vi "NAMEdll.vi"(7 "ln3":i32, 8 "error in (no error)":errorcluster, 9 "ln2":i32, 10 "ln1":i32, 11 "Mixure Cluster in":T1={"Mixture Name"="R410A", "Molecular weight (g/mol)"=72.5854142406597, "Critical temperature (K)"=343.606231592265, "Critical Pressure (kPa)"=4813.60652781276, "Critical Density (mol/L)"=0.0, "# Components"=2, "Fluid File Paths"=[path "C:/Program Files (x86)/National Instruments/LabVIEW 2015/user.lib/REFPROP/fluids/R32.FLD", path "C:/Program Files (x86)/National Instruments/LabVIEW 2015/user.lib/REFPROP/fluids/R125.FLD"], "Component molar fractions"=[0.697614699375863, 0.302385300624138], "Refprop Main Directory"=path "C:/Program Files (x86)/National Instruments/LabVIEW 2015/user.lib/REFPROP", "DLL Version Number"=0.0}) -> (0 "error out":errorcluster, 3 "name out":string)   [LabVIEW 2015]
doc: "subroutine NAMEdll(icomp, hnam, hn80, hcasn, hnam_length, hn80_length, hcasn_length)\nProvides name information for the specified component.\n\nINPUTS:\n icomp ::Component number in mixture; 1 for pure fluid\n ln1 :: length of variable hnam (default: 12)\n ln2 :: length of variable hn80 (default: 80)\n ln3 :: length of variable hcasn (default: 12)\n\nOUTPUTS:\nhnam :: Component name (character*12)\nhn80 :: Component name - long form (character*80) To return the file name used when SETUP\n was called (without path), send -icomp. If path is also needed, use PASSCMN.\nhcasn :: ID (Chemical Abstracts Service) number (character*12)"
uses:
  Ctl/Mixture Composition cluster_d.ctl
  REFPROP.dll
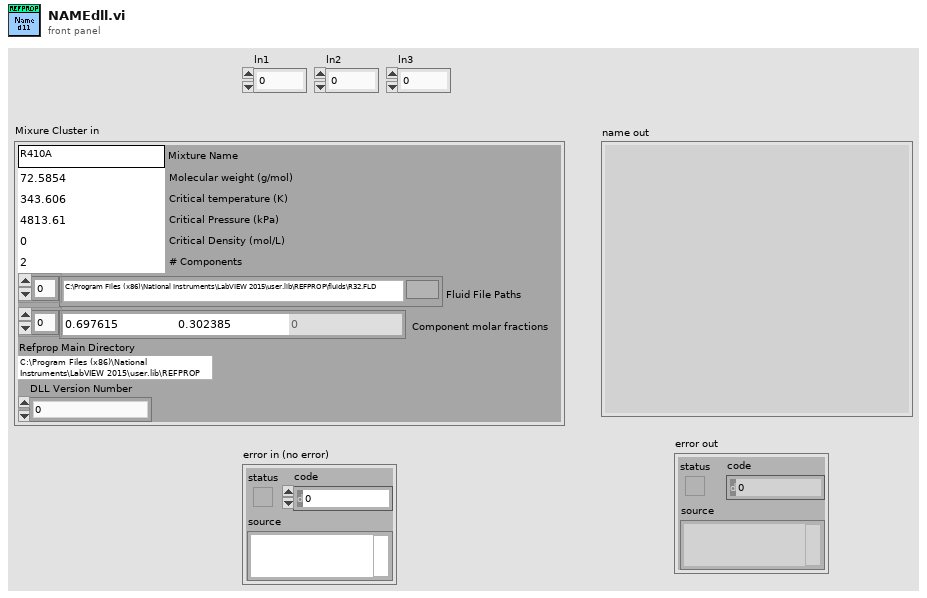
[diagram p1: front panel]
types:
  T1 = typedef "Mixture Composition cluster_d.ctl" = cluster{"Mixture Name":string, "Molecular weight (g/mol)":dbl, "Critical temperature (K)":dbl, "Critical Pressure (kPa)":dbl, "Critical Density (mol/L)":dbl, "# Components":i32, "Fluid File Paths":path[], "Component molar fractions":dbl[], "Refprop Main Directory":path, "DLL Version Number":dbl}
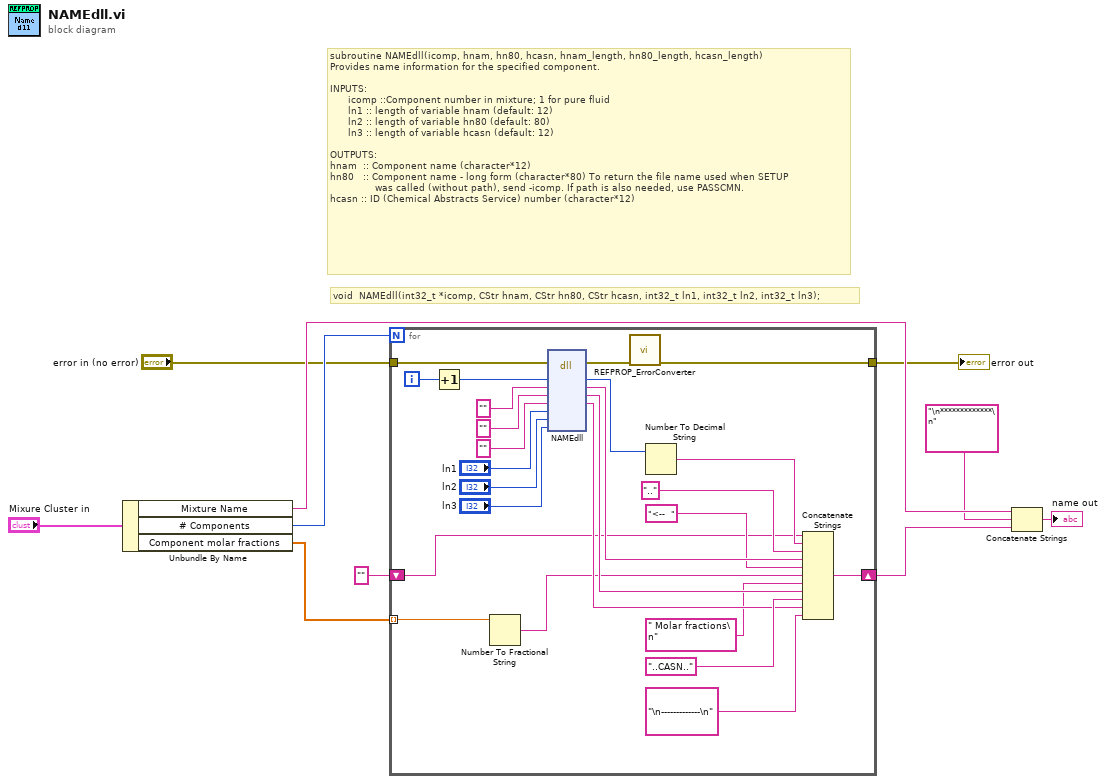
[diagram p0: block diagram]
diagram:
  # "subroutine NAMEdll(icomp, hnam, hn80, hcasn, hnam_length, hn80_length, hcasn_length)\nProvides name information for the specified component.\n\nINPUTS:\n      icomp ::Component number in mixture; 1 for pure fluid\n      ln1 :: length of variable hnam (default: 12)\n      ln2 :: length of variable hn80 (default: 80)\n      ln3 :: length of variable hcasn (default: 12)\n\nOUTPUTS:\nhnam  :: Component name (character*12)\nhn80   :: Component name - long form (character*80) To return the file name used when SETUP\n               was called (without path), send -icomp. If path is also needed, use PASSCMN.\nhcasn :: ID (Chemical Abstracts Service) number (character*12)"
  # "void  NAMEdll(int32_t *icomp, CStr hnam, CStr hn80, CStr hcasn, int32_t ln1, int32_t ln2, int32_t ln3);"
  n1 = Unbundle By Name("Mixure Cluster in") -> ("Mixture Name"=w6:string, "# Components"=w9:i32, "Component molar fractions"=w8:dbl[])
  n2 = for {
    N: w9 -> [_]
    tunnel: "error in (no error)" -> [w29]
    tunnel: [w27] -> w1
    shift-right: [w18] -> w5
    shift-left: "" -> [w11]
    tunnel: w8 -> [w14] mode=indexing
    i -> [w26]
    n3 = Increment(x=w26) -> (x+1=w25:i32)
    n4 = Number To Fractional String(number=w14) -> (F-format string=w12:string)  [unwired: 3 in]
    n5 = dll-call lib="C:/Users/lauria/Desktop/REFPROP 10 LabVIEW Wrapper BETA/REFPROP/REFPROP.*" fn="NAMEdll"(error in=w29, "icomp"=w25, "hnam"="", "hn80"="", "hcasn"="", "ln1"="ln1", "ln2"="ln2", "ln3"="ln3") -> (error out=w28:errorcluster, "icomp"=w24:i32, "hnam"=w22:string, "hn80"=w21:string, "hcasn"=w16:string)  [unwired: 6 in, 1 out]
    n6 = call "REFPROP_ErrorConverter.vi"("error in (no error)"=w28) -> ("error out"=w27:errorcluster)  [unwired: 10 in]
    n7 = Number To Decimal String(number=w24) -> (decimal integer string=w23:string)  [unwired: 1 in]
    n8 = Concatenate Strings(w11, w23, ".." ("字符串"), w22, "<--  " ("字符串"), w12, " Molar fractions\n" ("字符串"), w21, "..CASN.." ("字符串"), w16, "\n-------------\n" ("字符串")) -> (w18:string)
  }
  "error out" <- w1
  n9 = Concatenate Strings(w6, "\n*************\n" ("字符串"), w5) -> (→"name out":string)
